vi "Enable or Disable PCP controls.vi"(11 "error in (no error)":errorcluster) -> (15 "error out":errorcluster)   [LabVIEW 2011]
doc: "This VI enables or disables the PCP controls based on the digital values that are read. The disable property nodes will not be written unless the condition for disabling/enabling has been changed."
uses:
  Measurments Handling/Common/Variable List Common Digital.ctl
  Measurments Handling/Status Digitalish.ctl
  Controll refrence groups.ctl
  Tool/Variable List Tool Digital.ctl
  emi Lib/Basic/1 - GUI/Control tools/Private/emi_Control enable and visibility array.vi
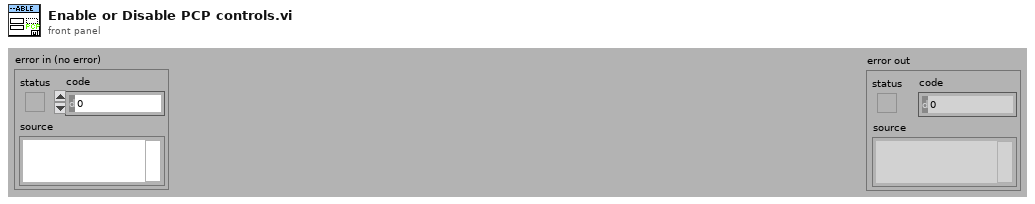
[diagram p1: front panel]
types:
  T1 = typedef "Variable List Tool Digital.ctl" = enum16{"Tool Error Controller", "Tool Stopped Controller", "Tool Relay 1", "Tool Relay 2", "Tool Both Relays", "Tool node Pressure 1", "Tool Error Pressure 1", "Tool Stopped Pressure 1", "Tool node Pressure 2", "Tool Error Pressure 2", "Tool Stopped Pressure 2", "Tool node Solenoid", "Tool Error Solenoid", "Tool Stopped Solenoid", "Tool Solenoid 1", "Tool Solenoid 2", "Tool Solenoid 3", "Tool node PSU", "Tool Error PSU", "Tool Stopped PSU", "Upper Tension Sub", "Tool Error Upper Tension Sub", "Tool Stopped Upper Tension Sub", "Lower Tension Sub", "Tool Error Lower Tension Sub", "Tool Stopped Lower Tension Sub", "Stroke Target seeking", "Stroke Moving Out", "Stroke Moving Inn", "Stroke valves set for Out", "Stroke valves set for In", "Stroke In (force)", "Stroke Out (force)", "Stroke Force decreasing(in)", "Stroke Force decreasing(out)", "Stroke Force change not correct", "Stroke SLIPS established P1", "Stroke SLIPS established P2", "Stroke SLIPS established", "Stroke Pressure Monitor Ongoing", "Stroke Pressure Monitor Ending ", "Tool Stroke enable Valve", "Tool Stroke direction Valve", "Tool Anchor Valve", "Stroker Var19 - Reserved", "Stroker Var20 - Reserved", "Stroker Var21 - Reserved", "Stroker Var22 - Reserved", "Stroker Var23 - Reserved", "Stroker Var24 - Reserved", "Tractor Var1 - Reserved", "Tractor Var2 - Reserved", "Tractor Var3 - Reserved", "Tractor Var4 - Reserved", "Tractor Var5 - Reserved", "Tractor Var6 - Reserved", "Tractor Var7 - Reserved", "Tractor Var8 - Reserved", "Oil filling mode", "Mill Bit Direction", "Position control", "Anchor", "Driller Var5 - Reserved", "Driller Var6 - Reserved", "Driller Var7 - Reserved", "Driller Var8 - Reserved"}
  T2 = typedef "Status Digitalish.ctl" = enum16{"NA", "False", "True"}
  T3 = typedef "Controll refrence groups.ctl" = enum16{"Controller. gen", "Controller . High G", "Stroker", "PCP Online", "PCP Local", "PCP HV On", "Driller", "Stroker Cmd Buttons", "Stroker Anchor Cmd Buttons", "Controller Relay Buttons", "PCP Start Telemetry", "PCP Start Motor", "Tractor", "Modem Status"}
  T4 = typedef "Variable List Common Digital.ctl" = enum16{"PCP Connected", "PCP PC Control", "HV PSU connected", "HV PSU HV Active", "Modem Connected", "Tool Connected", "CanBus interface"}
  T5 = cluster{"Controll collection":T3, bool, "State(Normal)":enum16{"Normal", "Disabled", "Grayed", "Hidden"}}
  T6 = cluster{"Controll collection":T3, bool, "State(Normal)":enum16{"Normal", "Disabled", "Grayed", "Hidden"}}[]
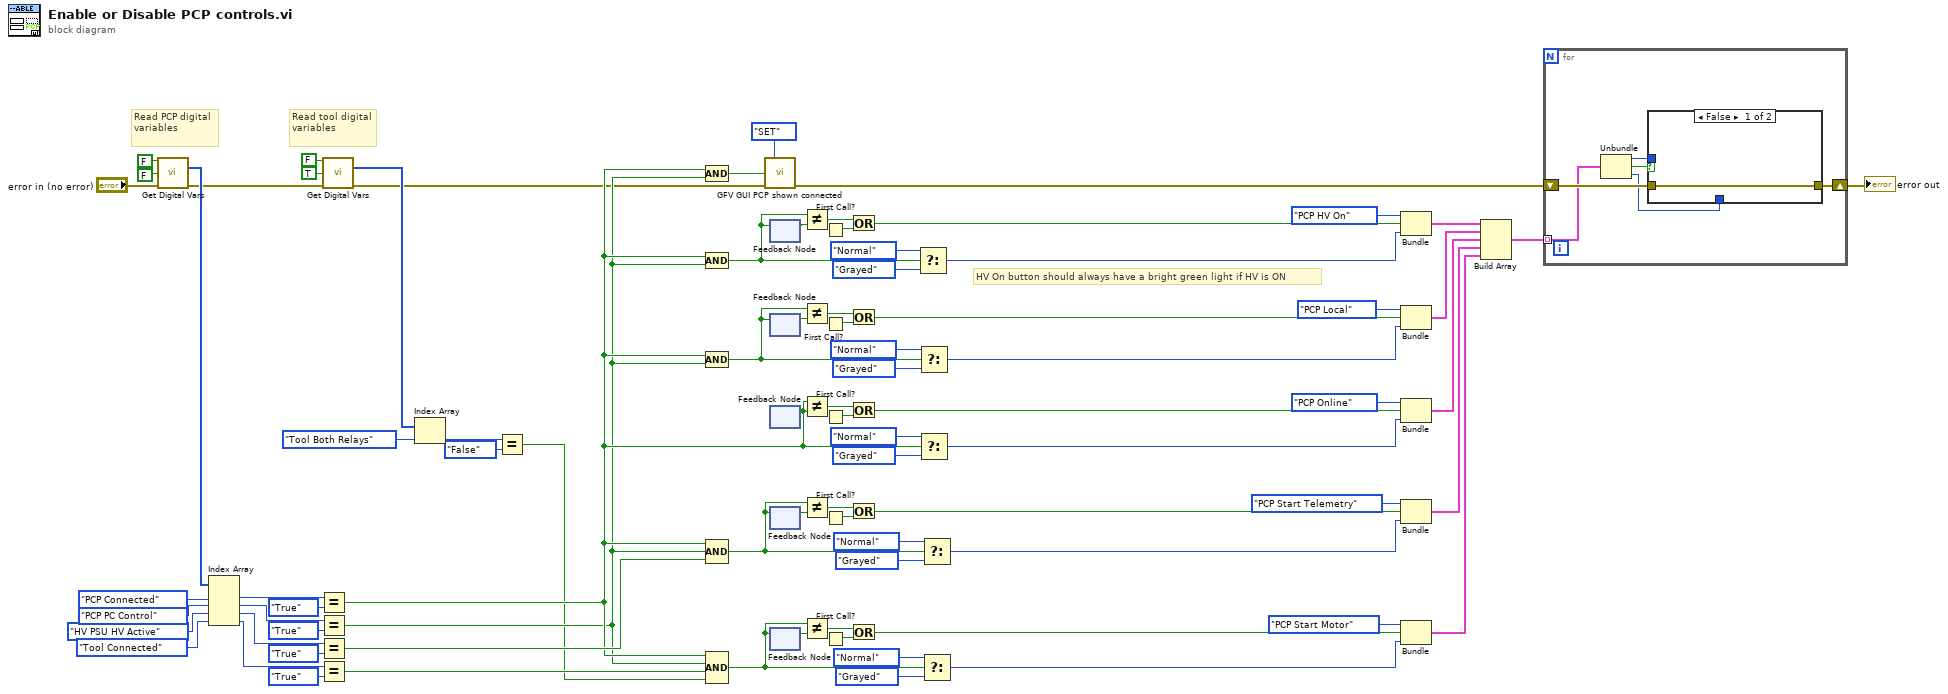
[diagram p0: block diagram]
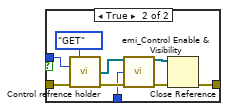
[diagram p2: hidden frame]
diagram:
  # "Read tool digital variables"
  # "Read PCP digital variables"
  # "HV On button should always have a bright green light if HV is ON"
  n1 = call "Get Digital Vars.vi"("Common alarm handling(F)"=FALSE, "Tool"=FALSE, "error in (no error)"="error in (no error)") -> ("Values"=w65:T2[], "error out"=w2:errorcluster)  [unwired: 6 in, 5 out]
  n2 = Index Array(array=w65, index #1=Variable_List_Common_Digital."PCP Connected" ("Action"), index #2=Variable_List_Common_Digital."PCP PC Control" ("Action"), index #3=Variable_List_Common_Digital."HV PSU HV Active" ("Action"), index #4=Variable_List_Common_Digital."Tool Connected" ("Action")) -> (element #1=w68:T2, element #2=w63:T2, element #3=w40:T2, element #4=w39:T2)
  n3 = Equal?(x=w68, y=Status_Digitalish."True") -> (x = y?=w10:bool)
  n4 = Equal?(x=w63, y=Status_Digitalish."True") -> (x = y?=w9:bool)
  n5 = Equal?(x=w40, y=Status_Digitalish."True") -> (x = y?=w13:bool)
  n6 = Equal?(x=w39, y=Status_Digitalish."True") -> (x = y?=w11:bool)
  n7 = call "Get Digital Vars.vi"("Common alarm handling(F)"=FALSE, "Tool"=TRUE, "error in (no error)"=w2) -> ("Values"=w7:T2[], "error out"=w6:errorcluster)  [unwired: 6 in, 5 out]
  n8 = Index Array(array=w7, index=Variable_List_Tool_Digital."Tool Both Relays") -> (element=w4:T2)
  n9 = Equal?(x=w4, y=Status_Digitalish."False") -> (x = y?=w3:bool)
  n10 = Compound Arithmetic op=AND(w10, w9) -> (w16:bool)
  n11 = Compound Arithmetic op=AND(w10, w9) -> (w15:bool)
  n12 = Compound Arithmetic op=AND(w10, w9) -> (w14:bool)
  n13 = Compound Arithmetic op=AND(w10, w9, w13) -> (w12:bool)
  n14 = Compound Arithmetic op=AND(w10, w9, w11, w3) -> (w8:bool)
  n15 = call "GFV GUI PCP shown connected.vi"("Action(GET)"=enum16{"GET", "SET"}."SET", "Shown connected in"=w16, "error in (no error)"=w6) -> ("error out"=w80:errorcluster)  [unwired: 11 in, 1 out]
  n16 = feedback #1() -> (w59:bool)  [unwired: 1 in]
  n17 = feedback-in #1(w15) -> ()
  n18 = feedback #2() -> (w54:bool)  [unwired: 1 in]
  n19 = feedback-in #2(w14) -> ()
  n20 = feedback #3() -> (w53:bool)  [unwired: 1 in]
  n21 = feedback-in #3(w10) -> ()
  n22 = feedback #4() -> (w48:bool)  [unwired: 1 in]
  n23 = feedback-in #4(w12) -> ()
  n24 = feedback #5() -> (w47:bool)  [unwired: 1 in]
  n25 = feedback-in #5(w8) -> ()
  n26 = Not Equal?(x=w15, y=w59) -> (x != y?=w57:bool)
  n27 = Not Equal?(x=w14, y=w54) -> (x != y?=w56:bool)
  n28 = Not Equal?(x=w10, y=w53) -> (x != y?=w51:bool)
  n29 = Not Equal?(x=w12, y=w48) -> (x != y?=w50:bool)
  n30 = Not Equal?(x=w8, y=w47) -> (x != y?=w45:bool)
  n31 = First Call?() -> (First Call?: T/F=w58:bool)
  n32 = First Call?() -> (First Call?: T/F=w55:bool)
  n33 = First Call?() -> (First Call?: T/F=w52:bool)
  n34 = First Call?() -> (First Call?: T/F=w49:bool)
  n35 = First Call?() -> (First Call?: T/F=w46:bool)
  n36 = Or(x=w57, y=w58) -> (x .or. y?=w38:bool)
  n37 = Or(x=w56, y=w55) -> (x .or. y?=w29:bool)
  n38 = Or(x=w51, y=w52) -> (x .or. y?=w27:bool)
  n39 = Or(x=w50, y=w49) -> (x .or. y?=w25:bool)
  n40 = Or(x=w45, y=w46) -> (x .or. y?=w23:bool)
  n41 = Select(t=enum16{"Normal", "Disabled", "Grayed", "Hidden"}."Normal" ("State(Normal)"), s=w15, f=enum16{"Normal", "Disabled", "Grayed", "Hidden"}."Grayed" ("State(Normal)")) -> (s? t:f=w36:enum16{"Normal", "Disabled", "Grayed", "Hidden"})
  n42 = Select(t=enum16{"Normal", "Disabled", "Grayed", "Hidden"}."Normal" ("State(Normal)"), s=w14, f=enum16{"Normal", "Disabled", "Grayed", "Hidden"}."Grayed" ("State(Normal)")) -> (s? t:f=w28:enum16{"Normal", "Disabled", "Grayed", "Hidden"})
  n43 = Select(t=enum16{"Normal", "Disabled", "Grayed", "Hidden"}."Normal" ("State(Normal)"), s=w10, f=enum16{"Normal", "Disabled", "Grayed", "Hidden"}."Grayed" ("State(Normal)")) -> (s? t:f=w26:enum16{"Normal", "Disabled", "Grayed", "Hidden"})
  n44 = Select(t=enum16{"Normal", "Disabled", "Grayed", "Hidden"}."Normal" ("State(Normal)"), s=w12, f=enum16{"Normal", "Disabled", "Grayed", "Hidden"}."Grayed" ("State(Normal)")) -> (s? t:f=w24:enum16{"Normal", "Disabled", "Grayed", "Hidden"})
  n45 = Select(t=enum16{"Normal", "Disabled", "Grayed", "Hidden"}."Normal" ("State(Normal)"), s=w8, f=enum16{"Normal", "Disabled", "Grayed", "Hidden"}."Grayed" ("State(Normal)")) -> (s? t:f=w22:enum16{"Normal", "Disabled", "Grayed", "Hidden"})
  n46 = Bundle("Controll collection"=Controll_refrence_groups."PCP HV On", w38, "State(Normal)"=w36) -> (w31:T5)  [unwired: 1 in]
  n47 = Bundle("Controll collection"=Controll_refrence_groups."PCP Local", w29, "State(Normal)"=w28) -> (w21:T5)  [unwired: 1 in]
  n48 = Bundle("Controll collection"=Controll_refrence_groups."PCP Online", w27, "State(Normal)"=w26) -> (w20:T5)  [unwired: 1 in]
  n49 = Bundle("Controll collection"=Controll_refrence_groups."PCP Start Telemetry", w25, "State(Normal)"=w24) -> (w19:T5)  [unwired: 1 in]
  n50 = Bundle("Controll collection"=Controll_refrence_groups."PCP Start Motor", w23, "State(Normal)"=w22) -> (w18:T5)  [unwired: 1 in]
  n51 = Build Array(w31, w21, w20, w19, w18) -> (w30:T6)
  n52 = for {
    tunnel: w30 -> [w88] mode=indexing
    shift-right: [w84] -> w17
    shift-left: w80 -> [w89]
    n53 = Unbundle(w88) -> ("Controll collection"=w87:T3, w86:bool, "State(Normal)"=w85:enum16{"Normal", "Disabled", "Grayed", "Hidden"})
    n54 = case shown="False" w86 {
      tunnel: w89 -> [w90 w95]
      tunnel: [w90 w94] -> w84
      tunnel: w87 -> [_ w93]
      tunnel: w85 -> [_ w92]
      frame False {
      }
      frame True {
        n55 = call "Control refrence holder.vi"("Action(GET)"=enum16{"GET", "SET"}."GET", "Controll collection"=w93, "error in (no error)"=w95) -> ("Controlls out"=w99:refnum<vi>[], "error out"=w98:errorcluster)  [unwired: 11 in]
        n56 = call-poly "emi_Control Enable & Visibility.vi"("Controls"=w99, "State(Normal)"=w92, "error in"=w98) -> ("Constrols out"=w96:refnum<vi>[], "error out"=w97:errorcluster)  [unwired: 11 in]
        n57 = Close Reference(reference=w96, error in (no error)=w97) -> (error out=w94:errorcluster)
      }
    }
  }
  "error out" <- w17
